vi "HH Scope Write Waveform.vi"(8 "error in":errorcluster, 11 "DI ADC in":T1={"FIFO Indexes"={"Write"={"Capture Enable"=-1, "Capture Event"=-1, "Capture Length"=-1}, "Read"={"Capture dt [s]"=-1}}, "HH ADC Data"={"Output Array"=[], "New Data"=FALSE}, "Waveform Data"=[], "Waveform Session"=refnum}) -> (0 "error out":errorcluster, 3 "DI ADC out":T1={"FIFO Indexes"={"Write"={"Capture Enable"=-1, "Capture Event"=-1, "Capture Length"=-1}, "Read"={"Capture dt [s]"=-1}}, "HH ADC Data"={"Output Array"=[], "New Data"=FALSE}, "Waveform Data"=[], "Waveform Session"=refnum})   [LabVIEW 2016, in "DCM Engine.lvlib"]
uses:
  DCM Engine.lvlib
  Shared/Types/HH Scope.ctl
  <vilib>/NI Veristand/Custom Device Waveform API/Multiple Waveforms Write (DBL)/Multiple Waveforms Write (DBL).lvclass
  C:/Program Files (x86)/National Instruments/LabVIEW 2016/vi.lib/NI Veristand/Custom Device Waveform API/Waveform Session.lvclass
  <vilib>/NI Veristand/Custom Device API/Waveform Data Reference.ctl
  <vilib>/NI Veristand/Custom Device Waveform API/Waveform Session.lvclass/Waveform Session.ctl
  <vilib>/NI Veristand/Custom Device Waveform API/Multiple Waveforms Write (DBL)/Multiple Waveforms Write (DBL).lvclass/Multiple Waveforms Write (DBL).ctl
  <vilib>/NI Veristand/Custom Device Waveform API/Internal Comm Classes/WPL Comm/WPL Comm (2D DBL)/WPL Comm (2D DBL).lvclass/WPL Comm (2D DBL).ctl
  <vilib>/NI Veristand/Custom Device Waveform API/Internal Comm Classes/WPL Comm/WPL Comm.lvclass/WPL Comm.ctl
  <vilib>/NI Veristand/Custom Device Waveform API/Multiple Waveforms Write (DBL)/NI VeriStand - Write Multiple Waveforms (DBL).vi
  <vilib>/NI Veristand/Custom Device Waveform API/Multiple Waveforms Write (DBL)/NI VeriStand - Start Multiple Waveforms (DBL).vi
  <vilib>/NI Veristand/Custom Device Waveform API/Read Sample offset DVR.vi
  <vilib>/NI Veristand/Custom Device Waveform API/Internal Comm Classes/WPL Comm/WPL Comm (2D DBL)/Comm_write 2d dbl.vi
  <vilib>/NI Veristand/Custom Device Waveform API/Check Write Size.vi
  <vilib>/NI Veristand/Custom Device Waveform API/Check Opened.vi
  <vilib>/NI Veristand/Custom Device Waveform API/Internal Comm Classes/WPL Comm/WPL_start dbl waveform.vi
  <vilib>/NI Veristand/Custom Device Waveform API/Internal Comm Classes/WPL Comm/Direct Send WPL Command.vi
  <vilib>/NI Veristand/Custom Device Waveform API/Internal Comm Classes/WPL Comm/Convert Q Error to Shutdown Error.vi
  <vilib>/NI Veristand/Custom Device Waveform API/Internal Comm Classes/WPL Comm/Set t0 on Variant.vi
  <vilib>/NI Veristand/Custom Device Waveform API/Internal Comm Classes/WPL Comm/Send WPL Command.vi
  <vilib>/NI Veristand/Custom Device Waveform API/Internal Comm Classes/WPL Comm/WPL Comm (2D DBL)/WPL Comm (2D DBL).lvclass
  C:/Program Files (x86)/National Instruments/LabVIEW 2016/vi.lib/NI Veristand/Custom Device Waveform API/Internal Comm Classes/WPL Comm/WPL Comm.lvclass
  <vilib>/Utility/error.llb/Error Cluster From Error Code.vi
  <vilib>/NI Veristand/Custom Device Waveform API/NI_VS Custom Device Waveform API.lvlib
  <vilib>/NI VeriStand/Custom Device API/Custom Device API.lvlib
  DCM Shared.lvlib
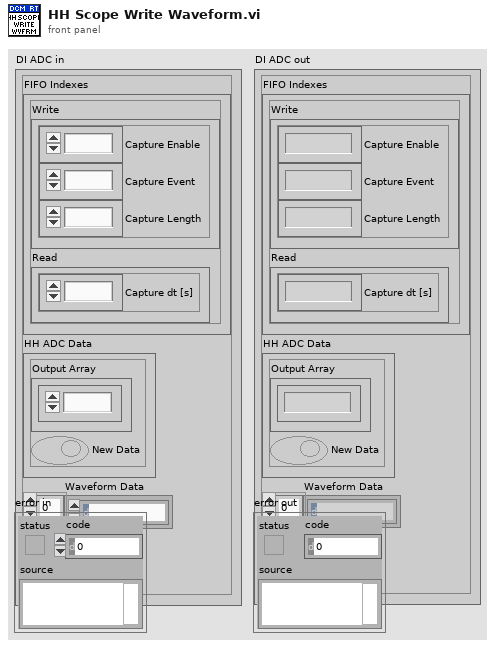
[diagram p1: front panel]
types:
  T1 = typedef "DCM Shared.lvlib/HH Scope.ctl" = cluster{"FIFO Indexes":cluster{"Write":cluster{"Capture Enable":i32, "Capture Event":i32, "Capture Length":i32}, "Read":cluster{"Capture dt [s]":i32}}, "HH ADC Data":cluster{"Output Array":sgl[][], "New Data":bool}, "Waveform Data":T2[], "Waveform Session":refnum<class "Multiple Waveforms Write (DBL).lvclass">}
  T2 = typedef "Custom Device API.lvlib/Waveform Data Reference.ctl" = i32
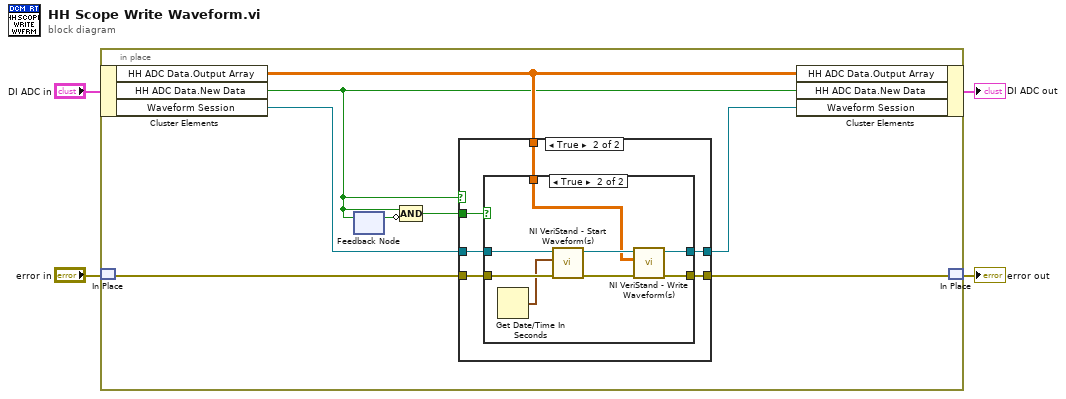
[diagram p0: block diagram]
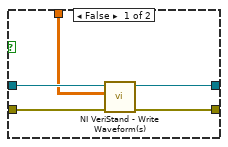
[diagram p3: hidden frame]
diagram:
  n1 = in-place {
    n2 = in-place-cluster #1("DI ADC in") -> ("HH ADC Data.Output Array"=w6:sgl[][], "HH ADC Data.New Data"=w5:bool, "Waveform Session"=w9:refnum<class "Multiple Waveforms Write (DBL).lvclass">)
    n3 = in-place-match #2("error in") -> (w12:errorcluster)
    n4 = feedback-in #3(w5) -> ()
    n5 = feedback #3() -> (w8:bool)  [unwired: 1 in]
    n6 = Compound Arithmetic op=AND(w5, invert w8) -> (w7:bool)
    n7 = case shown="True" w5 {
      tunnel: w9 -> [w13 w20]
      tunnel: [w13 w16] -> w10
      tunnel: w12 -> [w14 w19]
      tunnel: [w14 w18] -> w11
      tunnel: w7 -> [_ w17]
      tunnel: w6 -> [_ w15]
      frame False {
      }
      frame True {
        n8 = case shown="True" w17 {
          tunnel: w20 -> [w25 w28]
          tunnel: [w24 w33] -> w16
          tunnel: w19 -> [w22 w32]
          tunnel: [w23 w31] -> w18
          tunnel: w15 -> [w21 w26]
          frame False {
            n9 = call-poly <vilib>:"NI VeriStand - Write Waveform(s).vi"("error in (no error)"=w22, "Data"=w21, "Multiple Waveforms Write Session (DBL) in"=w25) -> ("error out"=w23:errorcluster, "Multiple Waveforms Write Session (DBL) out"=w24:refnum<class "Multiple Waveforms Write (DBL).lvclass">)  [unwired: 6 in, 1 out]
          }
          frame True {
            n10 = Get Date/Time In Seconds() -> (seconds since 1Jan1904=w27:timestamp)
            n11 = call-poly <vilib>:"NI VeriStand - Start Waveform(s).vi"("error in (no error)"=w32, "t0"=w27, "Multiple Waveforms Write Session (DBL) in"=w28) -> ("error out"=w29:errorcluster, "Multiple Waveforms Write Session (DBL) out"=w30:refnum<class "Multiple Waveforms Write (DBL).lvclass">)  [unwired: 7 in]
            n12 = call-poly <vilib>:"NI VeriStand - Write Waveform(s).vi"("error in (no error)"=w29, "Data"=w26, "Multiple Waveforms Write Session (DBL) in"=w30) -> ("error out"=w31:errorcluster, "Multiple Waveforms Write Session (DBL) out"=w33:refnum<class "Multiple Waveforms Write (DBL).lvclass">)  [unwired: 6 in, 1 out]
          }
        }
      }
    }
    n13 = in-place-cluster #1("HH ADC Data.Output Array"=w6, "HH ADC Data.New Data"=w5, "Waveform Session"=w10) -> (→"DI ADC out":T1)
    n14 = in-place-match #2(w11) -> (→"error out":errorcluster)
  }
